vi "Data_Header.vi"(8 "error in (no error)":errorcluster, 11 "ChirpEIS in":refnum<class "ChirpEIS.lvclass">) -> (0 "error out":errorcluster, 2 "Header String":string, 3 "ChirpEIS out":refnum<class "ChirpEIS.lvclass">)   [LabVIEW 2014, in "ChirpEIS.lvclass"]
uses:
  ChirpEIS.lvclass
  ChirpEIS.lvclass/ChirpEIS.ctl
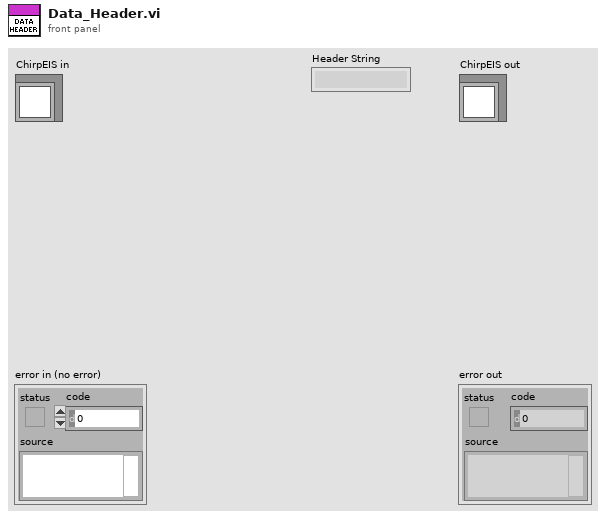
[diagram p1: front panel]
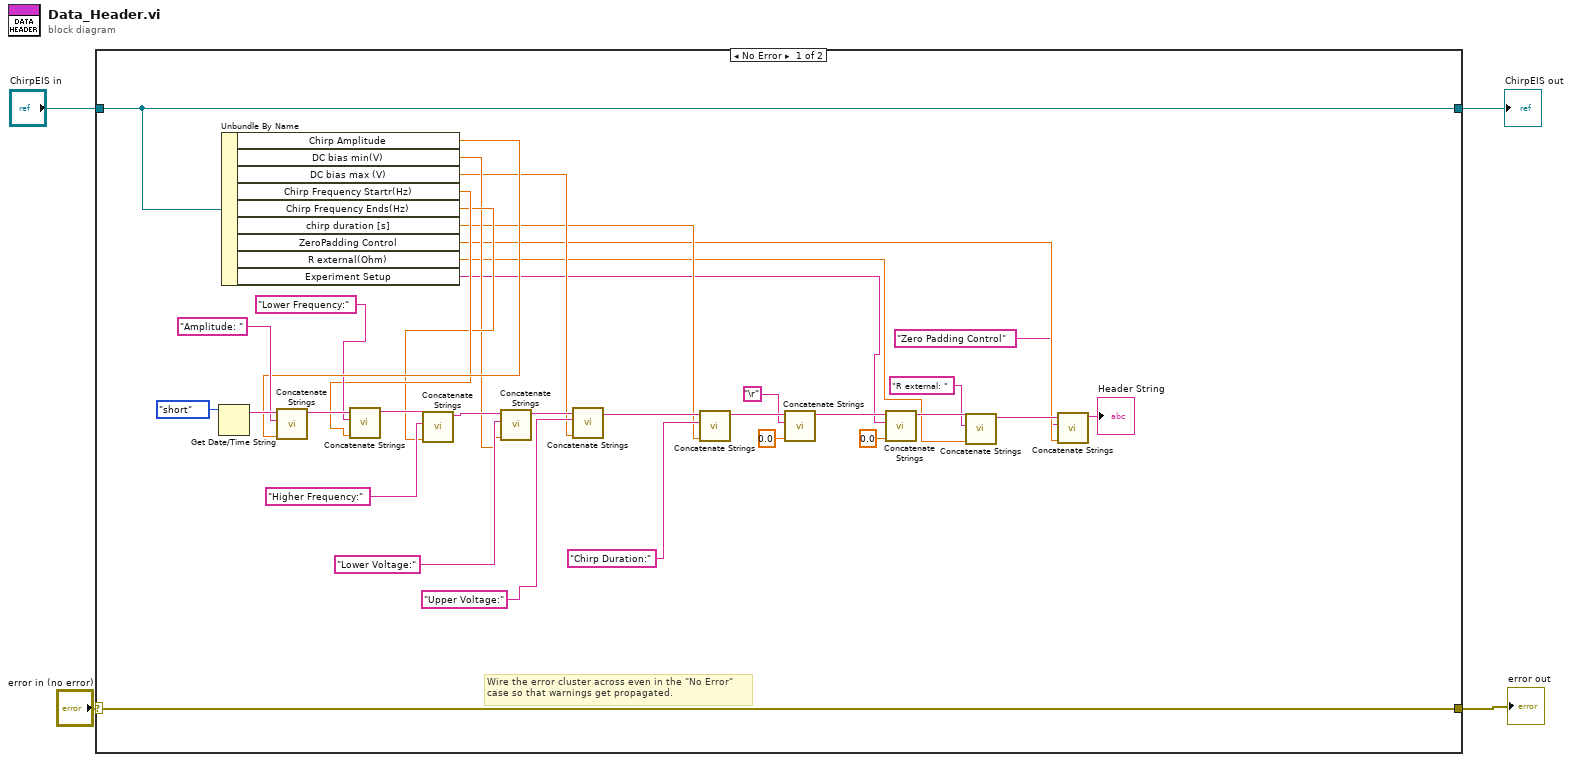
[diagram p0: block diagram]
diagram:
  n1 = case shown="No Error" "error in (no error)" {
    selector: "error in (no error)" -> [w38 w40]
    tunnel: [w38 w40] -> w3
    tunnel: [w35 w39] -> w1
    tunnel: "ChirpEIS in" -> [w35 w39]
    frame No Error {
      # "Wire the error cluster across even in the \"No Error\"\ncase so that warnings get propagated."
      n2 = Get Date/Time String(date format (0)=enum16{"short", "long", "abbreviated"}."short") -> (date string=w36:string)  [unwired: 2 in, 1 out]
      n3 = Unbundle By Name(w35) -> ("Chirp Amplitude"=w32:dbl, "DC bias min(V)"=w24:dbl, "DC bias max (V)"=w21:dbl, "Chirp Frequency Startr(Hz)"=w30:dbl, "Chirp Frequency Ends(Hz)"=w27:dbl, "chirp duration [s]"=w18:dbl, "ZeroPadding Control"=w7:dbl, "R external(Ohm)"=w9:dbl, "Experiment Setup"=w14:string)
      n4 = call "Concatenate Strings.vi"("Numeric In"=w32, "Description String"="Amplitude: " ("string"), "Previous String"=w36) -> ("Result String"=w34:string)  [unwired: 8 in]
      n5 = call "Concatenate Strings.vi"("Numeric In"=w30, "Description String"="Lower Frequency:" ("string"), "Previous String"=w34) -> ("Result String"=w29:string)  [unwired: 8 in]
      n6 = call "Concatenate Strings.vi"("Numeric In"=w27, "Description String"="Higher Frequency:" ("string"), "Previous String"=w29) -> ("Result String"=w26:string)  [unwired: 8 in]
      n7 = call "Concatenate Strings.vi"("Numeric In"=w24, "Description String"="Lower Voltage:" ("string"), "Previous String"=w26) -> ("Result String"=w23:string)  [unwired: 8 in]
      n8 = call "Concatenate Strings.vi"("Numeric In"=w21, "Description String"="Upper Voltage:" ("string"), "Previous String"=w23) -> ("Result String"=w19:string)  [unwired: 8 in]
      n9 = call "Concatenate Strings.vi"("Numeric In"=w18, "Description String"="Chirp Duration:" ("string"), "Previous String"=w19) -> ("Result String"=w17:string)  [unwired: 8 in]
      n10 = call "Concatenate Strings.vi"("Numeric In"=0.0, "Description String"="\r", "Previous String"=w17) -> ("Result String"=w15:string)  [unwired: 8 in]
      n11 = call "Concatenate Strings.vi"("Numeric In"=0.0, "Description String"=w14, "Previous String"=w15) -> ("Result String"=w11:string)  [unwired: 8 in]
      n12 = call "Concatenate Strings.vi"("Numeric In"=w9, "Description String"="R external: " ("string"), "Previous String"=w11) -> ("Result String"=w8:string)  [unwired: 8 in]
      n13 = call "Concatenate Strings.vi"("Numeric In"=w7, "Description String"="Zero Padding Control" ("string"), "Previous String"=w8) -> ("Result String"=→"Header String":string)  [unwired: 8 in]
    }
    frame Error {
    }
  }
  "error out" <- w3
  "ChirpEIS out" <- w1
